vi "ActionVIOnCompile.vi"(8 "error in (no error)":errorcluster, 11 "Device Item Ref in":T1 format="%.0x") -> (0 "error out":errorcluster)   [LabVIEW 2020, in "Communication Bus Template System Explorer.lvlib"]
uses:
  Communication Bus Template System Explorer.lvlib
  <vilib>/NI VeriStand/Custom Device API/Custom Device Item Ref.ctl
  Shared/Compiled.Settings.ctl
  <vilib>/NI VeriStand/Custom Device API/Data Reference.ctl
  <vilib>/NI VeriStand/Custom Device API/Block Data Reference.ctl
  Includes/Communication Bus Interfaces.lvlibp/Execution Unit/Execution Unit Factory/Execution Unit Factory.lvclass
  <vilib>/NI VeriStand/Custom Device Tools/Custom Device Utility Library/NI VeriStand - Search for Item by Name.vi
  <vilib>/NI VeriStand/Custom Device API/Set Item Property (Variant).vi
  <vilib>/NI VeriStand/Custom Device Tools/Custom Device Utility Library/Custom Device Utility Library.lvlib
  <vilib>/NI VeriStand/Custom Device API/Custom Device API.lvlib
  <vilib>/NI/NIVS Inline Async API/_Data Access System Explorer/Data Access System Explorer.lvlib
  Shared/Communication Bus Template Shared.lvlib
  Shared/Execution Unit Compiled Information.ctl
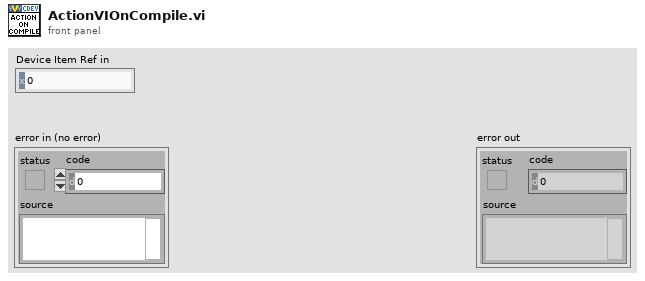
[diagram p1: front panel]
types:
  T1 = typedef "Custom Device API.lvlib/Custom Device Item Ref.ctl" = u64
  T2 = cluster{"Name":string, "Type":enum16{"Output/Write", "Input/Read", "Input/ReadWrite"}, "VS Refs":T1[]}
  T3 = enum16{"Output/Write", "Input/Read", "Input/ReadWrite"}
  T4 = typedef "Communication Bus Template Shared.lvlib/Compiled.Settings.ctl" = cluster{"Name":string, "Execution Unit Compiled Information":T5}
  T5 = typedef "Communication Bus Template Shared.lvlib/Execution Unit Compiled Information.ctl" = cluster{"Flattened Execution Unit":string, "Incoming Buffer":dbl[], "Outgoing Buffer":dbl[], "Incoming Data References":T6[], "Outgoing Data References":T7[]}
  T6 = typedef "Custom Device API.lvlib/Data Reference.ctl" = i32
  T7 = typedef "Custom Device API.lvlib/Block Data Reference.ctl" = cluster{"Data Reference":T6, "Offset":u64, "Length":u64}
  T8 = typedef "Custom Device API.lvlib/Custom Device Item Info.ctl" = cluster{"Name":string, "Is Channel":bool, "GUID":string, "Is Waveform":bool}
  T9 = typedef "Communication Bus Interfaces.lvlibp/Execution Unit.lvlib/Execution Unit Information.ctl" = cluster{"Execution Unit":refnum<class "Execution Unit.lvclass">, "Incoming Channels":T10[], "Outgoing Channels":T10[]}
  T10 = typedef "Communication Bus Interfaces.lvlibp/Custom Device API.lvlib/Custom Device Item Ref.ctl" = u64
  T11 = cluster{"Name":string, "Type":enum16{"Output/Write", "Input/Read", "Input/ReadWrite"}, "VS Refs":T1[]}[]
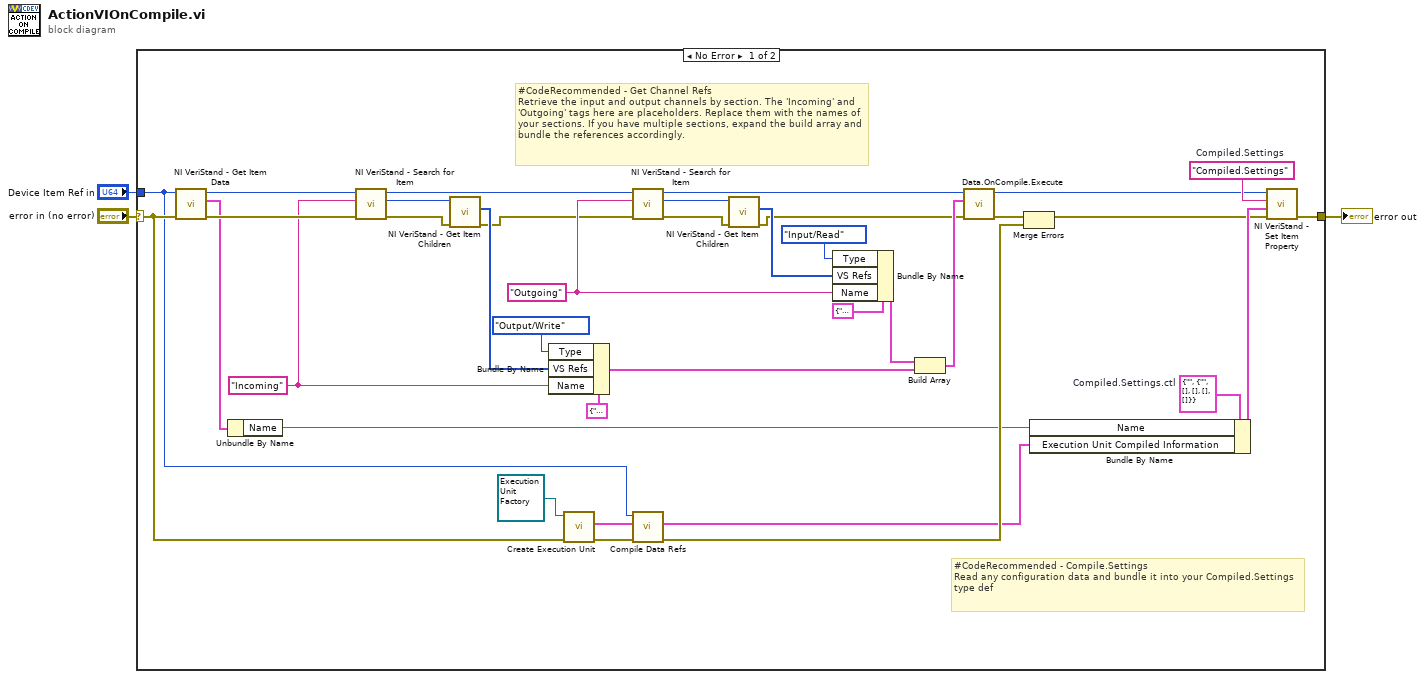
[diagram p0: block diagram]
diagram:
  n1 = case shown="No Error" "error in (no error)" {
    selector: "error in (no error)" -> [w11 w41]
    tunnel: [w34 w41] -> w2
    tunnel: "Device Item Ref in" -> [w9 _]
    frame No Error {
      w14 = T4 {"Name"="", "Execution Unit Compiled Information"={"Flattened Execution Unit"="", "Incoming Buffer"=[], "Outgoing Buffer"=[], "Incoming Data References"=[], "Outgoing Data References"=[]}}  # Compiled.Settings.ctl
      w28 = "Outgoing" ("Item Name")
      w30 = "Incoming" ("Item Name")
      w36 = "Compiled.Settings"  # Compiled.Settings
      # "#CodeRecommended - Get Channel Refs\nRetrieve the input and output channels by section. The 'Incoming' and 'Outgoing' tags here are placeholders. Replace them with the names of your sections. If you have multiple sections, expand the build array and bundle the references accordingly."
      # "#CodeRecommended - Compile.Settings\nRead any configuration data and bundle it into your Compiled.Settings type def"
      n2 = call <vilib>:"NI VeriStand - Get Item Data.vi"("error in (no error)"=w11, "Item Ref in"=w9) -> ("error out"=w32:errorcluster, "Item Info"=w31:T8, "Item Ref out"=w33:T1)  [unwired: 6 in, 1 out]
      n3 = Unbundle By Name(w31) -> ("Name"=w4:string)
      n4 = call-poly <vilib>:"NI VeriStand - Search for Item.vi"("error in"=w32, "Item Name"=w30, "Section Ref in"=w33) -> ("error out"=w40:errorcluster, "Item Ref"=w39:T1, "Section Ref out"=w17:T1)  [unwired: 5 in, 1 out]
      n5 = call <vilib>:"NI VeriStand - Get Item Children.vi"("error in (no error)"=w40, "Item Ref in"=w39) -> ("error out"=w16:errorcluster, "Child Refs"=w29:T1[])  [unwired: 6 in, 2 out]
      n6 = Bundle By Name(cluster=T2 {"Name"="", "Type"=enum."Output/Write", "VS Refs"=[]} ("Group"), "Type"=T3."Output/Write", "VS Refs"=w29, "Name"=w30) -> (w20:T2)
      n7 = call-dynamic "Create Execution Unit.vi"("error in"=w11, "Execution Unit Factory in"=refnum<class "Execution Unit Factory.lvclass"> refnum ("Communication Bus Template Interfaces:Execution Unit.lvlib:Execution Unit Factory.lvclass")) -> ("error out"=w10:errorcluster, "Execution Unit Information"=w12:T9)  [unwired: 7 in, 1 out]
      n8 = call-poly <vilib>:"NI VeriStand - Search for Item.vi"("error in"=w16, "Item Name"=w28, "Section Ref in"=w17) -> ("error out"=w37:errorcluster, "Item Ref"=w38:T1, "Section Ref out"=w18:T1)  [unwired: 5 in, 1 out]
      n9 = call "Compile Data Refs.vi"("error in"=w10, "Execution Unit Information"=w12, "Device Ref in"=w9) -> ("error out"=w6:errorcluster, "Execution Unit Compiled Information"=w5:T5)  [unwired: 6 in, 1 out]
      n10 = call <vilib>:"NI VeriStand - Get Item Children.vi"("error in (no error)"=w37, "Item Ref in"=w38) -> ("error out"=w19:errorcluster, "Child Refs"=w24:T1[])  [unwired: 6 in, 2 out]
      n11 = Bundle By Name(cluster=T2 {"Name"="", "Type"=enum."Output/Write", "VS Refs"=[]} ("Group"), "Type"=T3."Input/Read", "VS Refs"=w24, "Name"=w28) -> (w26:T2)
      n12 = Build Array(w26, w20) -> (w23:T11)
      n13 = call <vilib>:"Data.OnCompile.Execute.vi"("error in"=w19, "VS Ref Groups"=w23, "Custom Device Ref"=w18) -> ("error out"=w8:errorcluster, "Custom Device Ref"=w15:T1)  [unwired: 7 in]
      n14 = Merge Errors(w8, w6) -> (w7:errorcluster)
      n15 = Bundle By Name(cluster=w14, "Name"=w4, "Execution Unit Compiled Information"=w5) -> (w35:T4)
      n16 = call-poly <vilib>:"NI VeriStand - Set Item Property.vi"("error in (no error)"=w7, "Value"=w35, "Property Name"=w36, "Item Ref in"=w15) -> ("error out"=w34:errorcluster)  [unwired: 5 in, 2 out]
    }
    frame Error {
    }
  }
  "error out" <- w2
